vi "ErrorHandle.vi"(1 "Error":errorcluster[](array[cluster])) -> (0 "error IO":errorcluster caption="error out")   [LabVIEW 2018]
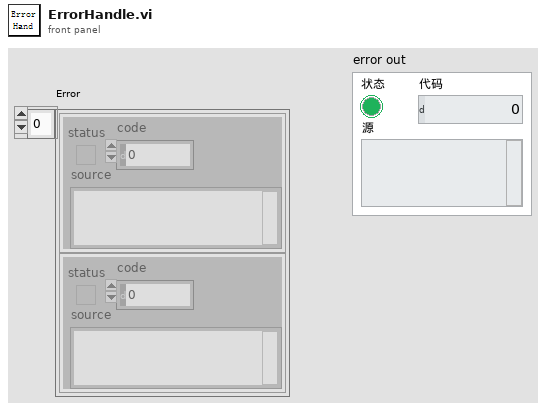
[diagram p1: front panel]
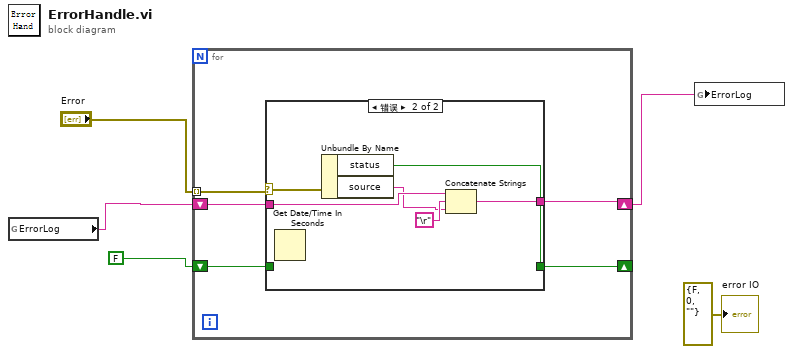
[diagram p0: block diagram]
diagram:
  n1 = global read "参数.vi" "ErrorLog"() -> (w3:string)
  n2 = for {
    tunnel: "Error" -> [w10] mode=indexing
    shift-right: [w9] -> _
    shift-left: FALSE -> [w8]
    shift-right: [w6] -> w2
    shift-left: w3 -> [w7]
    n3 = case shown="错误" w10 {
      selector: w10 -> [_ w18]
      tunnel: [w12 w17] -> w9
      tunnel: w8 -> [w12 _]
      tunnel: w7 -> [w11 w16]
      tunnel: [w11 w13] -> w6
      frame No Error {
      }
      frame Error {
        n4 = Get Date/Time In Seconds() -> ()  [unwired: 1 out]
        n5 = Unbundle By Name(w18) -> ("status"=w17:bool, "source"=w14:string)
        n6 = Concatenate Strings(w16, "\r", w14) -> (w13:string)
      }
    }
  }
  n7 = global write "参数.vi" "ErrorLog"(w2) -> ()
  "error IO" <- errorcluster {"status"=FALSE, "code"=0, "source"=""} ("error IO")
